vi "Write Image File.vi"(8 "Error in at file creation":errorcluster, 10 "Image to write":T1, 11 "File path for writing the file":path=path "C:/Users/user/Desktop/Studienarbeit Image Processing/LabView Learnings/Test Images/IMGABinary.jpg") -> (0 "Error out at image file writing":errorcluster, 3 "Image Out after file writing":T1)   [LabVIEW 2016]
uses:
  <vilib>/vision/Image Controls.llb/IMAQ Image.ctl
panel:
  # "VI to write an image file"
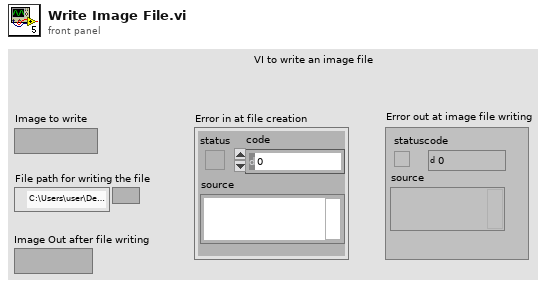
[diagram p1: front panel]
types:
  T1 = typedef "IMAQ Image.ctl" = refnum<image>
  T2 = enum16{"open", "replace", "create", "open or create", "replace or create", "replace or create with confirmation"}
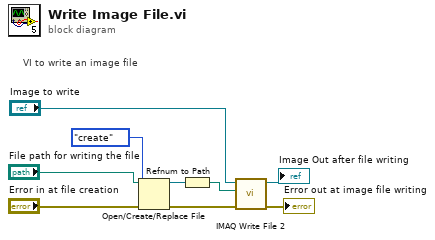
[diagram p0: block diagram]
diagram:
  # "VI to write an image file"
  n1 = Open/Create/Replace File(file path (use dialog)="File path for writing the file", error in="Error in at file creation", operation (0:open)=T2."create") -> (refnum out=w6:refnum<file>, error out=w7:errorcluster)  [unwired: 3 in, 1 out]
  n2 = Refnum to Path(1:w6) -> (0:w5:path)
  n3 = call-poly "IMAQ Write File 2"("error in (no error)"=w7, "File Path"=w5, "Image"="Image to write") -> ("error out"=→"Error out at image file writing":errorcluster, "Image Out (duplicate)"=→"Image Out after file writing":T1)  [unwired: 7 in]
